vi "获取实例.vi"() -> (3 "data value reference":refnum<data-value>)   [LabVIEW 2011, in "单例.lvlib"]
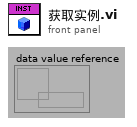
[diagram p1: front panel]
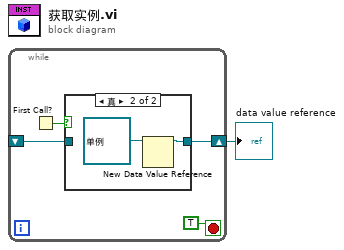
[diagram p0: block diagram]
diagram:
  n1 = while {
    shift-right: [w3] -> w1
    shift-left: _ -> [w2]
    stop <- TRUE stop-if-true
    n2 = First Call?() -> (First Call?: T/F=w5:bool)
    n3 = case shown="真" w5 {
      tunnel: [w6 w7] -> w3
      tunnel: w2 -> [w6 _]
      frame False {
      }
      frame True {
        n4 = New Data Value Reference(data value=refnum<class "单例.lvclass"> refnum ("单例.lvlib:单例.lvclass")) -> (data value reference=w7:refnum<data-value>)  [unwired: 1 in, 1 out]
      }
    }
  }
  "data value reference" <- w1
